vi "Set Bucket Notification Configuration.vi"(4 "Region":T1, 7 "NotificationConfiguration":T2, 8 "error in (no error)":errorcluster, 9 "Bucket":string) -> (0 "error out":errorcluster, 3 "Test message ID":string)   [LabVIEW 2015, in "LV Interface for Amazon S3.lvlib"]
doc: "This operation <B>enables/disables notifications of specified events</B> for a bucket. If the bucket owner is the same as the resource being notified, the bucket owner has permission to publish notifications to the topic by default. Otherwise, the owner of the topic must create a policy to enable the bucket owner to publish to the topic. By default, <B>only the bucket owner can configure notifications</B> on a bucket. However, bucket <B>owners can</B> use a bucket policy to <B>grant permission to other users to set this configuration with s3:PutBucketNotification permission</B>. After you call this operation to configure notifications on a bucket, Amazon S3 publishes a test notification to ensure that the resource exists and that the bucket owner has permission to publish. If the notification is successfully published, the operation updates the bucket configuration and returns the message ID of the test notification sent."
uses:
  LV Interface for Amazon S3.lvlib
  Typedefs/AMZ_S3_NotificationConfiguration.ctl
  Typedefs/AMZ_S3_CompleteTopicConfiguration.ctl
  Typedefs/AMZ_S3_Event.ctl
  Typedefs/AMZ_S3_FilterRule.ctl
  Typedefs/AMZ_S3_CloudFunctionConfiguration.ctl
  Typedefs/AMZ_S3_QueueConfiguration.ctl
  Typedefs/AMZ_S3_LocationConstraint.ctl
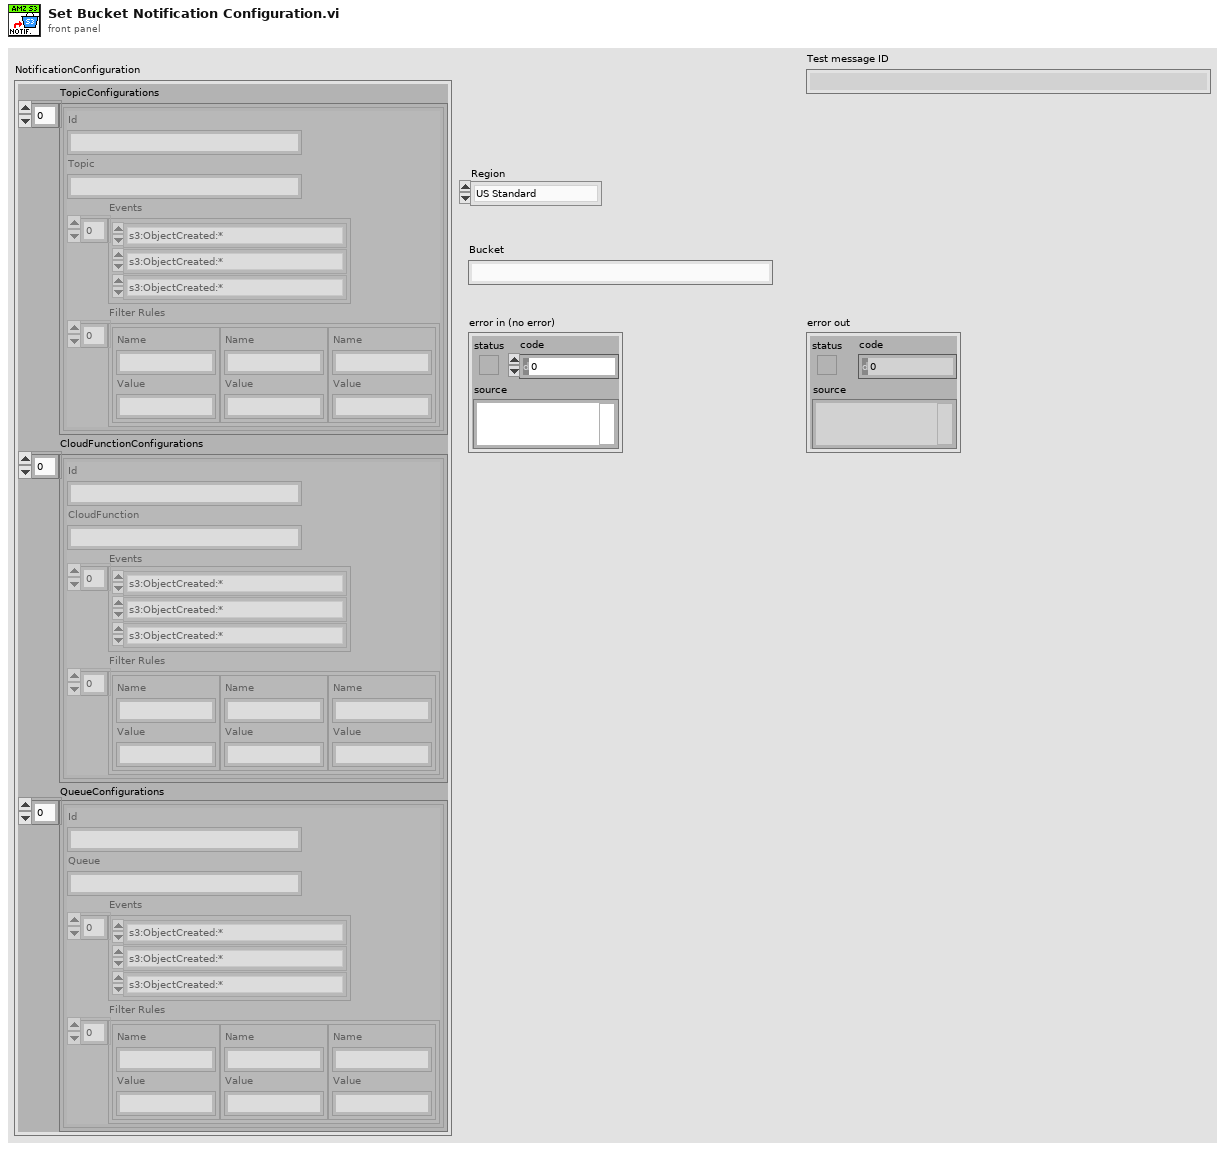
[diagram p1: front panel]
types:
  T1 = typedef "LV Interface for Amazon S3.lvlib/AMZ_S3_LocationConstraint.ctl" = enum16{"US Standard", "us-east-2", "us-west-1", "us-west-2", "ap-northeast-1", "ap-northeast-2", "ap-southeast-1", "ap-southeast-2", "ca-central-1", "eu-central-1", "eu-west-1", "eu-west-2", "sa-east-1"}
  T2 = typedef "LV Interface for Amazon S3.lvlib/AMZ_S3_NotificationConfiguration.ctl" = cluster{"TopicConfigurations":T3[], "CloudFunctionConfigurations":T6[], "QueueConfigurations":T7[]}
  T3 = typedef "LV Interface for Amazon S3.lvlib/AMZ_S3_CompleteTopicConfiguration.ctl" = cluster{"Id":string, "Topic":string, "Events":T4[], "Filter Rules":T5[]}
  T4 = typedef "LV Interface for Amazon S3.lvlib/AMZ_S3_Event.ctl" = enum16{"s3:ObjectCreated:*", "s3:ObjectCreated:Put", "s3:ObjectCreated:Post", "s3:ObjectCreated:Copy", "s3:ObjectCreated:CompleteMultipartUpload", "s3:ObjectRemoved:*", "s3:ObjectRemoved:Delete", "s3:ObjectRemoved:DeleteMarkerCreated", "s3:ReducedRedundancyLostObject"}
  T5 = typedef "LV Interface for Amazon S3.lvlib/AMZ_S3_FilterRule.ctl" = cluster{"Name":string, "Value":string}
  T6 = typedef "LV Interface for Amazon S3.lvlib/AMZ_S3_CloudFunctionConfiguration.ctl" = cluster{"Id":string, "CloudFunction":string, "Events":T4[], "Filter Rules":T5[]}
  T7 = typedef "LV Interface for Amazon S3.lvlib/AMZ_S3_QueueConfiguration.ctl" = cluster{"Id":string, "Queue":string, "Events":T4[], "Filter Rules":T5[]}
  T8 = typedef "LV Interface for Amazon S3.lvlib/AMZ_S3_Call Results.ctl" = enum16{"Success", "UndefinedError", "AccessDenied", "AccountProblem", "AmbiguousGrantByEmailAddress", "BadDigest", "BucketAlreadyExists", "BucketAlreadyOwnedByYou", "BucketNotEmpty", "CredentialsNotSupported", "CrossLocationLoggingProhibited", "EntityTooSmall", "EntityTooLarge", "ExpiredToken", "IllegalVersioningConfigurationException", "IncompleteBody", "IncorrectNumberOfFilesInPostRequest", "InlineDataTooLarge", "InternalError", "InvalidAccessKeyId", "InvalidAddressingHeader", "InvalidArgument", "InvalidBucketName", "InvalidDigest", "InvalidLocationConstraint", "InvalidPart", "InvalidPartOrder", "InvalidPayer", "InvalidPolicyDocument", "InvalidRange", "InvalidSecurity", "InvalidSOAPRequest", "InvalidStorageClass", "InvalidTargetBucketForLogging", "InvalidToken", "InvalidURI", "KeyTooLong", "MalformedACLError", "MalformedPOSTRequest", "MalformedXML", "MaxMessageLengthExceeded", "MaxPostPreDataLengthExceededError", "MetadataTooLarge", "MethodNotAllowed", "MissingAttachment", "MissingContentLength", "MissingRequestBodyError", "MissingSecurityElement", "MissingSecurityHeader", "NoLoggingStatusForKey", "NoSuchBucket", "NoSuchKey", "NoSuchUpload", "NoSuchVersion", "NotImplemented", "NotSignedUp", "OperationAborted", "PermanentRedirect", "PreconditionFailed", "Redirect", "RequestIsNotMultiPartContent", "RequestTimeout", "RequestTimeTooSkewed", "RequestTorrentOfBucketError", "SignatureDoesNotMatch", "SlowDown", "TemporaryRedirect", "TokenRefreshRequired", "TooManyBuckets", "UnexpectedContent", "UnresolvableGrantByEmailAddress", "UserKeyMustBeSpecified", "LabVIEWError"}
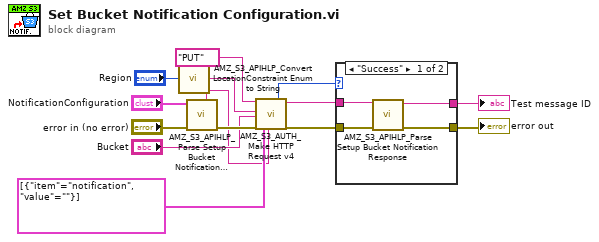
[diagram p0: block diagram]
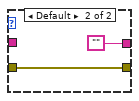
[diagram p2: hidden frame]
diagram:
  n1 = call "AMZ_S3_APIHLP_Convert LocationConstraint Enum to String.vi"("Location"="Region") -> ("Location String"=w1:string)  [unwired: 4 in]
  n2 = call "AMZ_S3_APIHLP_Parse Setup Bucket Notification Request Parameters.vi"("error in (no error)"="error in (no error)", "Setup Notification Request parameters"="NotificationConfiguration") -> ("error out"=w10:errorcluster, "PUT Data"=w3:string)  [unwired: 8 in]
  n3 = call "AMZ_S3_AUTH_Make HTTP Request v4.vi"("HTTP-Verb"="PUT", "Region"=w1, "Bucket"="Bucket", "error in"=w10, "request parameters"=cluster{"item":string, "value":string}[] [{"item"="notification", "value"=""}], "request body"=w3) -> ("Call Result"=w8:T8, "response headers"=w7:string, "error out"=w9:errorcluster)  [unwired: 10 in, 1 out]
  n4 = case shown="\"Success\"" w8 {
    tunnel: w9 -> [w18 w20]
    tunnel: w7 -> [w17 _]
    tunnel: [w16 ""] -> w11
    tunnel: [w15 w20] -> w12
    frame "Success" {
      n5 = call "AMZ_S3_APIHLP_Parse Setup Bucket Notification Response.vi"("error in (no error)"=w18, "Response header"=w17) -> ("error out"=w15:errorcluster, "Test message id"=w16:string)  [unwired: 8 in]
    }
    frame Default {
    }
  }
  "Test message ID" <- w11
  "error out" <- w12
